vi "coax cable time delays.vi"(1 "channel":u8) -> (0 "Coax cable time (x32ps)":u64)   [LabVIEW 2016]
uses:
  Global Variables/Global Resolution.vi
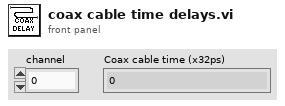
[diagram p1: front panel]
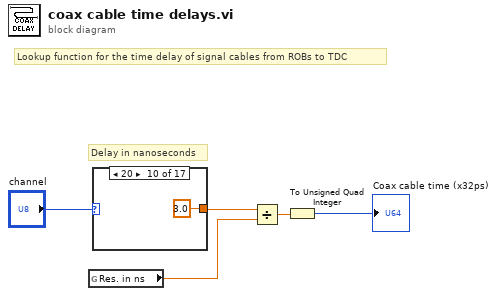
[diagram p0: block diagram]
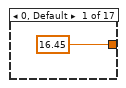
[diagram p2: hidden frame]
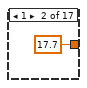
[diagram p3: hidden frame]
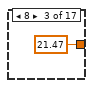
[diagram p4: hidden frame]
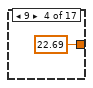
[diagram p5: hidden frame]
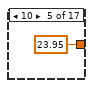
[diagram p6: hidden frame]
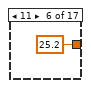
[diagram p7: hidden frame]
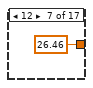
[diagram p8: hidden frame]
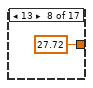
[diagram p9: hidden frame]
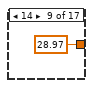
[diagram p10: hidden frame]
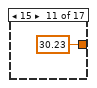
[diagram p11: hidden frame]
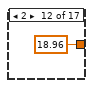
[diagram p12: hidden frame]
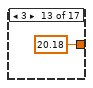
[diagram p13: hidden frame]
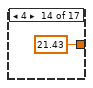
[diagram p14: hidden frame]
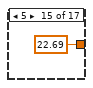
[diagram p15: hidden frame]
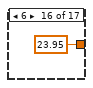
[diagram p16: hidden frame]
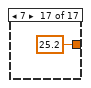
[diagram p17: hidden frame]
diagram:
  # "Delay in nanoseconds"
  # "Lookup function for the time delay of signal cables from ROBs to TDC"
  n1 = global read "Global Resolution.vi" "Res. in ns"() -> (w3:ext)
  n2 = case shown="20" "channel" {
    tunnel: [16.45 17.7 21.47 22.69 23.95 25.2 26.46 27.72 28.97 3.0 30.23 18.96 20.18 21.43 22.69 23.95 25.2] -> w4
    frame 0, Default {
    }
    frame 1 {
    }
    frame 8 {
    }
    frame 9 {
    }
    frame 10 {
    }
    frame 11 {
    }
    frame 12 {
    }
    frame 13 {
    }
    frame 14 {
    }
    frame 20 {
    }
    frame 15 {
    }
    frame 2 {
    }
    frame 3 {
    }
    frame 4 {
    }
    frame 5 {
    }
    frame 6 {
    }
    frame 7 {
    }
  }
  n3 = Divide(x=w4, y=w3) -> (x/y=w2:ext)
  n4 = To Unsigned Quad Integer(1:w2) -> (0:→"Coax cable time (x32ps)":u64)
